vi "Configure Trigger (Ethernet - Basic).vi"(0 "VISA resource name":refnum<visa-resource-name>, 1 "Qualifier (0: Less Than)":u16(ring) items=["Less Than", "More Than", "Equal", "Unequal", "More Equal", "In Range", "Out Range"], 5 "Trigger Source (9: Bus 1)":u16(ring)=9 items=["Bus 1"=9, "Bus 2"=10], 7 "Frame Type (0: Basic)":u16(ring) items=["Basic", "Q-Tag"], 9 "Condition (0: SFD)":u16(ring) items=["SFD", "MAC Address", "MAC Length", "Data", "EOP", "Idle", "FCS Error", "IP Header", "TCP Header", "Q-Tag"], 11 "error in (no error)":errorcluster) -> (4 "VISA resource name out":refnum<visa-resource-name>, 15 "error out":errorcluster)   [LabVIEW 2016, in "Tektronix DPO MSO 2000 4000 Series.lvlib"]
doc: "Configures Ethernet trigger basic settings.\n\n<B>Note:</B>\nThis VI only applies to DPO4034B, DPO4054B, DPO4104B, MSO4034B, MSO4054B, MSO4104B."
uses:
  Tektronix DPO MSO 2000 4000 Series.lvlib
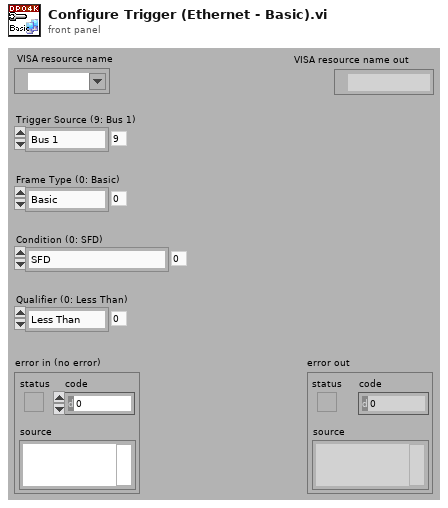
[diagram p1: front panel]
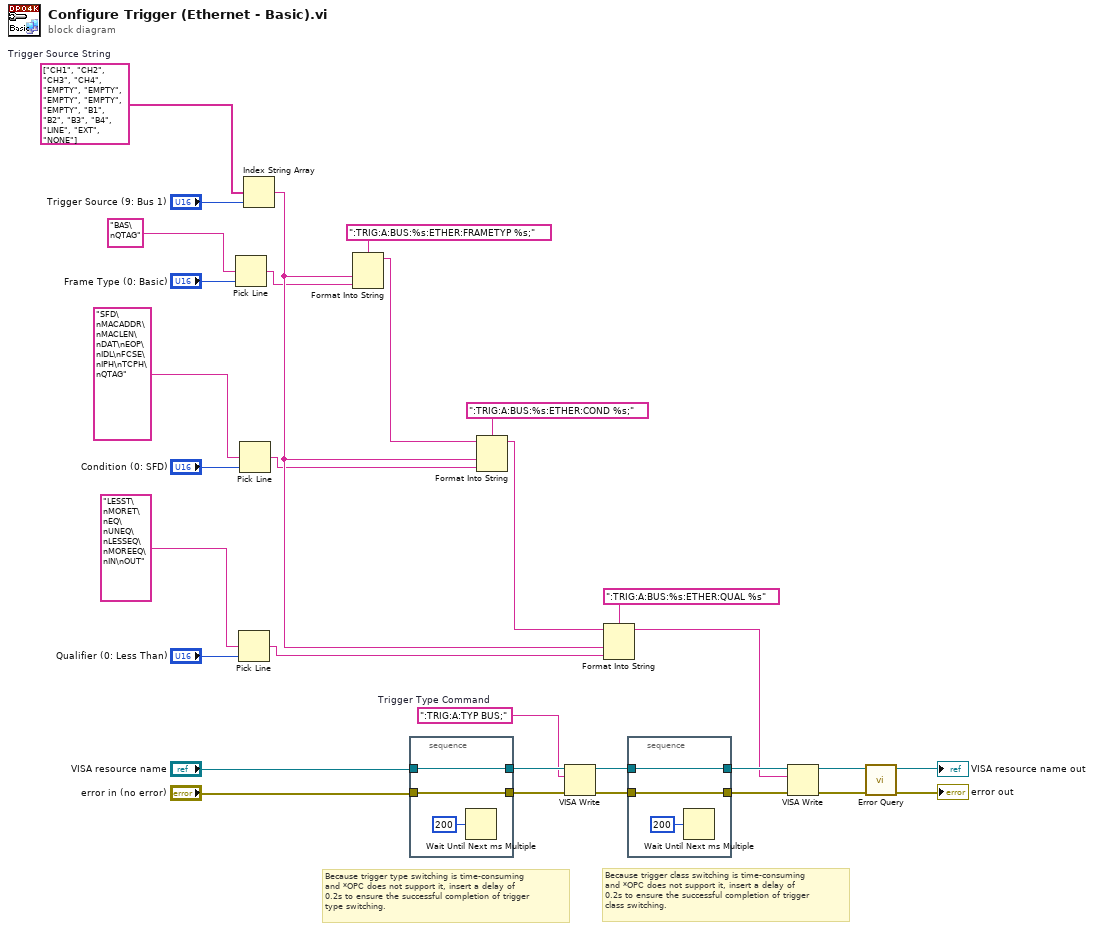
[diagram p0: block diagram]
diagram:
  w24 = string[] ["CH1", "CH2", "CH3", "CH4", "EMPTY", "EMPTY", "EMPTY", "EMPTY", "EMPTY", "B1", "B2", "B3", "B4", "LINE", "EXT", "NONE"]  # Trigger Source String
  w29 = ":TRIG:A:TYP BUS;"  # Trigger Type Command
  # "Because trigger class switching is time-consuming\nand *OPC does not support it, insert a delay of\n0.2s to ensure the successful completion of trigger\nclass switching."
  # "Because trigger type switching is time-consuming\nand *OPC does not support it, insert a delay of\n0.2s to ensure the successful completion of trigger\ntype switching."
  n1 = Pick Line(multi-line string="BAS\nQTAG", line index="Frame Type (0: Basic)") -> (output string=w10:string)  [unwired: 1 in]
  n2 = Pick Line(multi-line string="LESST\nMORET\nEQ\nUNEQ\nLESSEQ\nMOREEQ\nIN\nOUT", line index="Qualifier (0: Less Than)") -> (output string=w4:string)  [unwired: 1 in]
  n3 = Pick Line(multi-line string="SFD\nMACADDR\nMACLEN\nDAT\nEOP\nIDL\nFCSE\nIPH\nTCPH\nQTAG", line index="Condition (0: SFD)") -> (output string=w7:string)  [unwired: 1 in]
  n4 = Index String Array(1:"Trigger Source (9: Bus 1)", 2:w24) -> (0:w13:string)  [unwired: 1 in]
  n5 = Format Into String(format string=":TRIG:A:BUS:%s:ETHER:FRAMETYP %s;", w13, w10) -> (resulting string=w2:string)  [unwired: 2 in, 1 out]
  n6 = stacked-sequence {
    tunnel: "VISA resource name" -> [w33]
    tunnel: [w33] -> w31
    tunnel: "error in (no error)" -> [w32]
    tunnel: [w32] -> w30
    frame #0 {
      n7 = Wait Until Next ms Multiple(millisecond multiple=u32 200) -> ()  [unwired: 1 out]
    }
  }
  n8 = Format Into String(format string=":TRIG:A:BUS:%s:ETHER:COND %s;", initial string=w2, w13, w7) -> (resulting string=w3:string)  [unwired: 1 in, 1 out]
  n9 = VISA Write(VISA resource name=w31, write buffer=w29, error in (no error)=w30) -> (VISA resource name out=w28:refnum<visa-resource-name>, error out=w27:errorcluster)  [unwired: 1 out]
  n10 = Format Into String(format string=":TRIG:A:BUS:%s:ETHER:QUAL %s", initial string=w3, w13, w4) -> (resulting string=w1:string)  [unwired: 1 in, 1 out]
  n11 = stacked-sequence {
    tunnel: w28 -> [w36]
    tunnel: [w36] -> w26
    tunnel: w27 -> [w35]
    tunnel: [w35] -> w25
    frame #0 {
      n12 = Wait Until Next ms Multiple(millisecond multiple=u32 200) -> ()  [unwired: 1 out]
    }
  }
  n13 = VISA Write(VISA resource name=w26, write buffer=w1, error in (no error)=w25) -> (VISA resource name out=w22:refnum<visa-resource-name>, error out=w21:errorcluster)  [unwired: 1 out]
  n14 = call "Error Query.vi"("error in (no error)"=w21, "VISA resource name"=w22) -> ("error out"=→"error out":errorcluster, "VISA resource name out"=→"VISA resource name out":refnum<visa-resource-name>)  [unwired: 6 in, 2 out]
